vi "Read.vi"(8 "error in (no error)":errorcluster, 9 "timeout ms (25000)":i32, 10 "# bytes to read":i32, 11 "Socket in":refnum<class "Socket.lvclass">) -> (0 "error out":errorcluster, 1 "timed out?":bool, 2 "Read Bytes":u8[](array[numeric]), 3 "Socket out":refnum<class "Socket.lvclass">)   [LabVIEW 2021, in "Sockets.lvlib" / "Socket.lvclass"]
doc: "Reads data from a socket connection.\nWebSockets 2.0.1.40\nSam Sharp - MediaMongrels Ltd\nCopyright (c) 2019, MediaMongrels Ltd"
uses:
  Socket.lvclass
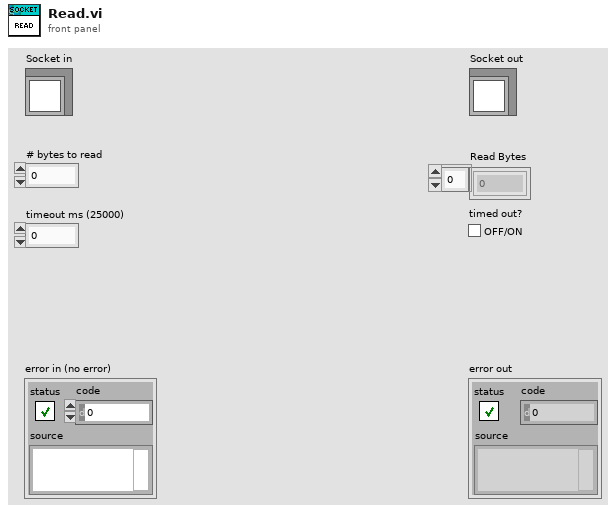
[diagram p1: front panel]
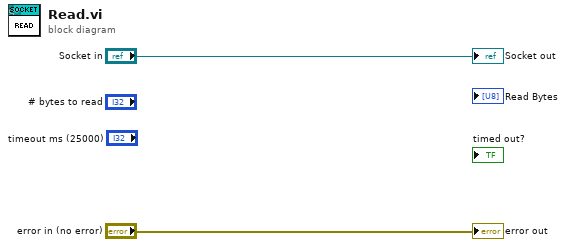
[diagram p0: block diagram]
diagram:
  "error out" <- "error in (no error)"
  "Socket out" <- "Socket in"
